vi "Multipart request - simple.vi"() -> ()   [LabVIEW 2015]
uses:
  <vilib>/addons/zeromq/socket_type.ctl
  <vilib>/addons/zeromq/zmq_context.lvclass
  <vilib>/addons/zeromq/zmq_socket.lvclass
  <vilib>/addons/zeromq/zeromq.lvlib
panel:
  in  "Delay before reconnect (mS)":u32=1000
  in  "transmit queue limit":i32=3
  out "transmit queue size":i32
  out "data received":string[](array[string])
  out "data sent":string[](array[string])=["", "0"]
  in  "1st frame":string="Test"
  out "error out":errorcluster
  in  "stop":bool
  in  "endpoint":string="tcp://127.0.0.1:5555"
  # "ZeroMQ Multipart request VI - simple"
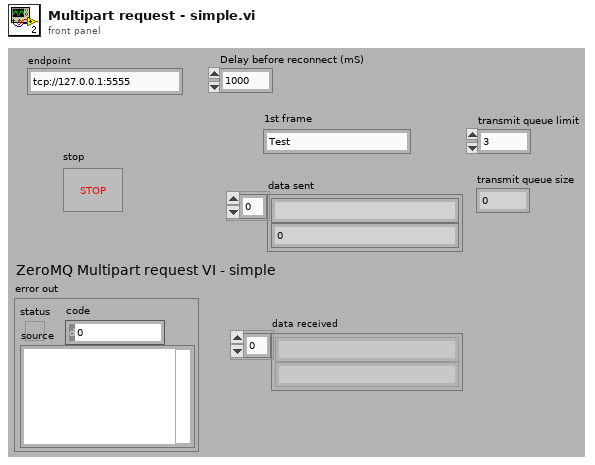
[diagram p1: front panel]
types:
  T1 = typedef "zeromq.lvlib/socket_type.ctl" = enum8{"ZMQ_PAIR", "ZMQ_PUB", "ZMQ_SUB", "ZMQ_REQ", "ZMQ_REP", "ZMQ_DEALER", "ZMQ_ROUTER", "ZMQ_PULL", "ZMQ_PUSH", "ZMQ_XPUB", "ZMQ_XSUB"}
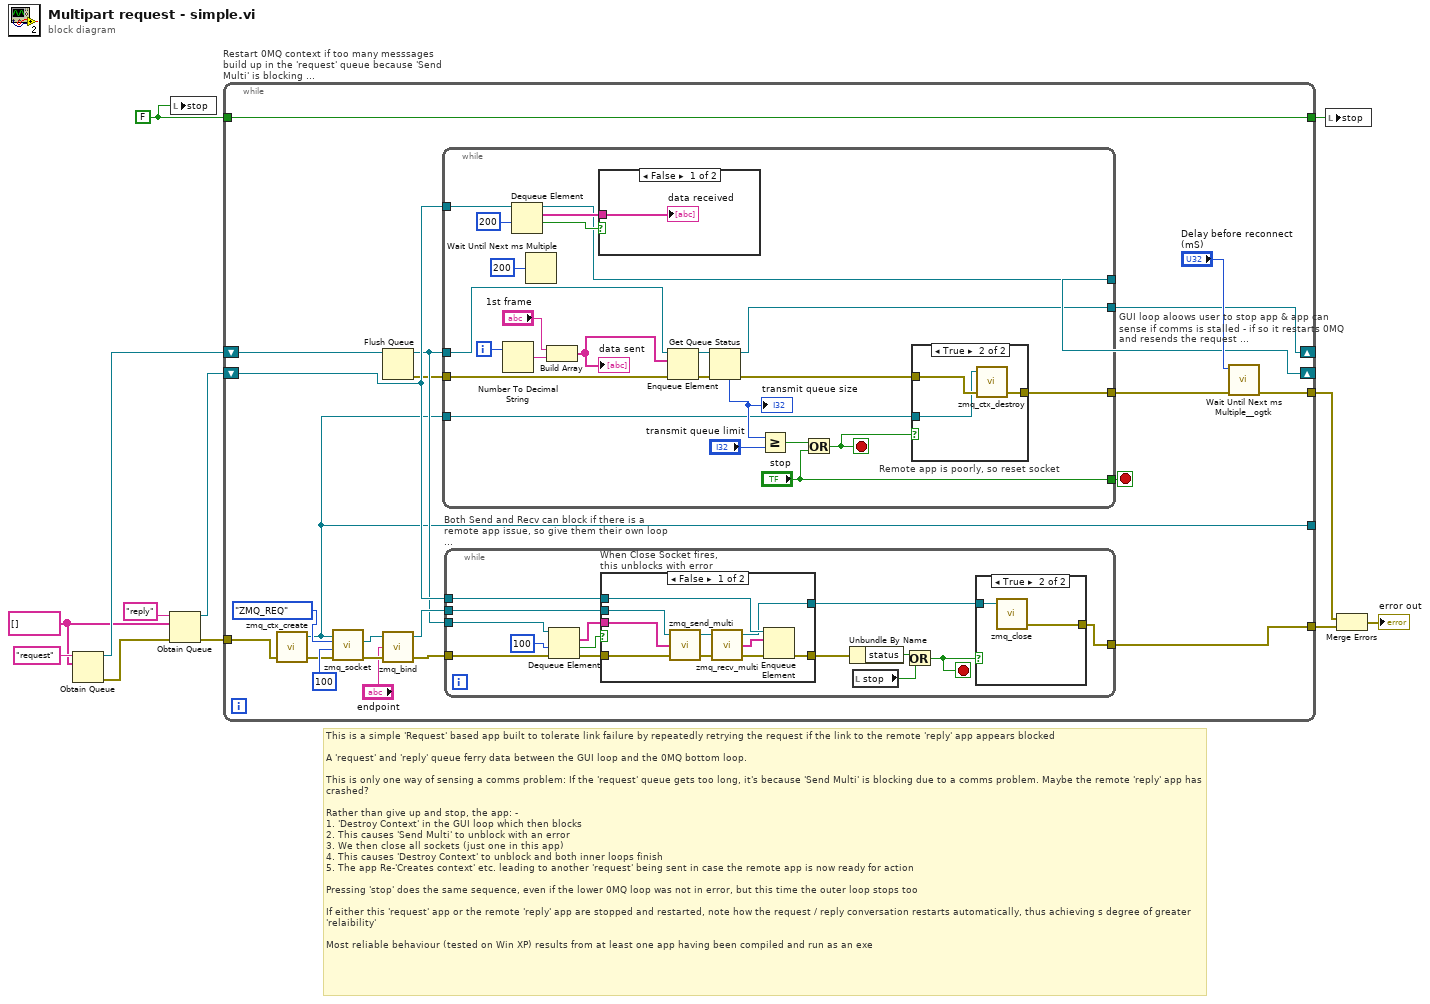
[diagram p0: block diagram]
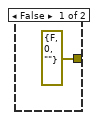
[diagram p4: hidden frame]
diagram:
  w4 = FALSE ("stop")
  w10 = string[] []
  # "This is a simple 'Request' based app built to tolerate link failure by repeatedly retrying the request if the link to the remote 'reply' app appears blocked\n\nA 'request' and 'reply' queue ferry data between the GUI loop and the 0MQ bottom loop.\n\nThis is only one way of sensing a comms problem: If the 'request' queue gets too long, it's because 'Send Multi' is blocking due to a comms problem. Maybe the remote 'reply' app has crashed? \n\nRather than give up and stop, the app: -\n1. 'Destroy Context' in the GUI loop which then blocks\n2. This causes 'Send Multi' to unblock with an error\n3. We then close all sockets (just one in this app)\n4. This causes 'Destroy Context' to unblock and both inner loops finish\n5. The app Re-'Creates context' etc. leading to another 'request' being sent in case the remote app is now ready for action\n\nPressing 'stop' does the same sequence, even if the lower 0MQ loop was not in error, but this time the outer loop stops too\n\nIf either this 'request' app or the remote 'reply' app are stopped and restarted, note how the request / reply conversation restarts automatically, thus achieving s degree of greater 'relaibility' \n\nMost reliable behaviour (tested on Win XP) results from at least one app having been compiled and run as an exe"
  n1 = Obtain Queue(name (unnamed)="request", element data type=w10) -> (queue out=w12:refnum<queue>, error out=w8:errorcluster)  [unwired: 3 in, 1 out]
  n2 = Obtain Queue(name (unnamed)="reply", element data type=w10, error in (no error)=w8) -> (queue out=w7:refnum<queue>, error out=w6:errorcluster)  [unwired: 2 in, 1 out]
  n3 = local write "stop"(w4) -> ()
  n4 = while "Restart 0MQ context if too many messsages build up in the 'request' queue because 'Send Multi' is blocking ..." {
    tunnel: w6 -> [w20]
    shift-right: [w27] -> _
    shift-left: w12 -> [w24]
    shift-right: [w26] -> _
    shift-left: w7 -> [w28]
    tunnel: [w18] -> _
    tunnel: w4 -> [w17]
    tunnel: [w17] -> w5
    tunnel: [w15] -> w3
    tunnel: [w14] -> w2
    stop <- w16 stop-if-true
    n5 = call <vilib>:"zmq_ctx_create.vi"("error in"=w20) -> ("error out"=w19:errorcluster, "context out"=w18:refnum<class "zmq_context.lvclass">)  [unwired: 3 in]
    n6 = call <vilib>:"zmq_socket.vi"("error in"=w19, "linger (ms)"=100, "socket type"=socket_type."ZMQ_REQ", "context in"=w18) -> ("error out"=w34:errorcluster, "socket out"=w13:refnum<class "zmq_socket.lvclass">)  [unwired: 1 in, 1 out]
    n7 = Flush Queue(queue=w24) -> (queue out=w23:refnum<queue>, error out=w22:errorcluster)  [unwired: 1 in, 1 out]
    n8 = call <vilib>:"zmq_bind.vi"("error in"=w34, "endpoint"="endpoint", "socket in"=w13) -> ("error out"=w25:errorcluster, "socket out"=w30:refnum<class "zmq_socket.lvclass">)  [unwired: 1 in]
    n9 = while "GUI loop aloows user to stop app & app can sense if comms is stalled - if so it restarts 0MQ and resends the request ..." {
      tunnel: w23 -> [w54]
      tunnel: w28 -> [w53]
      tunnel: ["stop"] -> w16
      tunnel: [w40] -> w27
      tunnel: [w39] -> w26
      tunnel: w22 -> [w38]
      tunnel: [w37] -> w21
      tunnel: w18 -> [w35]
      i -> [w55]
      stop <- w43 stop-if-true
      n10 = Number To Decimal String(number=w55) -> (decimal integer string=w57:string)  [unwired: 1 in]
      n11 = Dequeue Element(queue=w53, timeout in ms (-1)=200) -> (queue out=w39:refnum<queue>, element=w52:string[], timed out?=w51:bool)  [unwired: 1 in, 1 out]
      n12 = Wait Until Next ms Multiple(millisecond multiple=u32 200) -> ()  [unwired: 1 out]
      n13 = Build Array("1st frame", w57) -> (w48:string[])
      "data sent" <- w48
      n14 = case shown="False" w51 {
        tunnel: w52 -> [w58 _]
        frame False {
          "data received" <- w58
        }
        frame True {
        }
      }
      n15 = Enqueue Element(queue=w54, element=w48, error in (no error)=w38) -> (queue out=w46:refnum<queue>, error out=w47:errorcluster)  [unwired: 1 in, 1 out]
      n16 = Get Queue Status(queue=w46, error in (no error)=w47) -> (queue out=w40:refnum<queue>, error out=w36:errorcluster, # elements in queue=w45:i32)  [unwired: 1 in, 5 out]
      "transmit queue size" <- w45
      n17 = Greater Or Equal?(x=w45, y="transmit queue limit") -> (x >= y?=w42:bool)
      n18 = Or(x=w42, y="stop") -> (x .or. y?=w43:bool)
      n19 = case "Remote app is poorly, so reset socket" shown="True" w43 {
        tunnel: [w59 w62] -> w37
        tunnel: w36 -> [w59 w61]
        tunnel: w35 -> [_ w60]
        frame False {
        }
        frame True {
          n20 = call <vilib>:"zmq_ctx_destroy.vi"("error in"=w61, "context in"=w60) -> ("error out"=w62:errorcluster)  [unwired: 3 in]
        }
      }
    }
    n21 = while "Both Send and Recv can block if there is a remote app issue, so give them their own loop ..." {
      tunnel: w30 -> [w76]
      tunnel: w23 -> [w73]
      tunnel: w28 -> [w70]
      tunnel: w25 -> [w69]
      tunnel: [w64] -> w15
      stop <- w63 stop-if-true
      n22 = Dequeue Element(queue=w73, timeout in ms (-1)=100, error in (no error)=w69) -> (element=w74:string[], timed out?=w75:bool, error out=w71:errorcluster)  [unwired: 1 out]
      n23 = case "When Close Socket fires,  this unblocks with error" shown="False" w75 {
        tunnel: w71 -> [w89 w91]
        tunnel: [w82 w91] -> w65
        tunnel: w76 -> [w86 w90]
        tunnel: w74 -> [w85 _]
        tunnel: w70 -> [w84 _]
        tunnel: [w80 w90] -> w68
        frame False {
          n24 = call <vilib>:"zmq_send_multi.vi"("error in"=w89, "parts"=w85, "socket in"=w86) -> ("error out"=w87:errorcluster, "socket out"=w88:refnum<class "zmq_socket.lvclass">)  [unwired: 1 in]
          n25 = call <vilib>:"zmq_recv_multi.vi"("error in"=w87, "socket in"=w88) -> ("error out"=w83:errorcluster, "parts"=w81:string[], "socket out"=w80:refnum<class "zmq_socket.lvclass">)  [unwired: 1 in]
          n26 = Enqueue Element(queue=w84, element=w81, error in (no error)=w83) -> (error out=w82:errorcluster)  [unwired: 1 in, 2 out]
        }
        frame True {
        }
      }
      n27 = Unbundle By Name(w65) -> ("status"=w67:bool)
      n28 = local read "stop"() -> (w66:bool)
      n29 = Or(x=w67, y=w66) -> (x .or. y?=w63:bool)
      n30 = case shown="True" w63 {
        tunnel: [errorcluster {"status"=FALSE, "code"=0, "source"=""} ("error out") w79] -> w64
        tunnel: w68 -> [_ w78]
        frame False {
        }
        frame True {
          n31 = call <vilib>:"zmq_close.vi"("socket"=w78) -> ("error out"=w79:errorcluster)  [unwired: 4 in]
        }
      }
    }
    n32 = call <userlib>:"Wait Until Next ms Multiple__ogtk.vi"("error in (no error)"=w21, "milliseconds to wait"="Delay before reconnect (mS)") -> ("error out"=w14:errorcluster)  [unwired: 8 in, 1 out]
  }
  n33 = local write "stop"(w5) -> ()
  n34 = Merge Errors(w2, w3) -> (→"error out":errorcluster)
